vi "UV_Parameters.vi"(6 "A/M (F:auto)":bool, 7 "R/W (F:read)":bool, 8 "error in":errorcluster, 9 "param":T1, 10 "CHN":T2 items=["All", "CH1", "CH2", "CH3", "CH4"], 11 "VISA resource":refnum<visa-resource-name>) -> (0 "error out":errorcluster, 2 "chn param":u8[](array[numeric]) format="%.0x", 3 "VISA resource out":refnum<visa-resource-name>, 5 "Err?":bool)   [LabVIEW 8.6]
uses:
  TypeDef/UVLed_func.ctl
  TypeDef/UVLed_channel.ctl
panel:
  # "For Manual and Auto Mode Only"
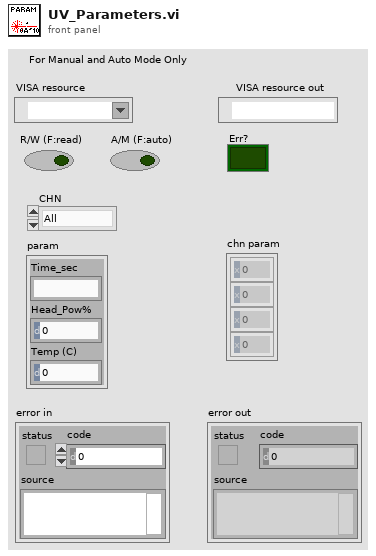
[diagram p1: front panel]
types:
  T1 = cluster{"Time_sec":string, "Head_Pow%":i32, "Temp (C)":u8}
  T2 = typedef "UVLed_channel.ctl" = u16
  T3 = typedef "UVLed_func.ctl" = u16
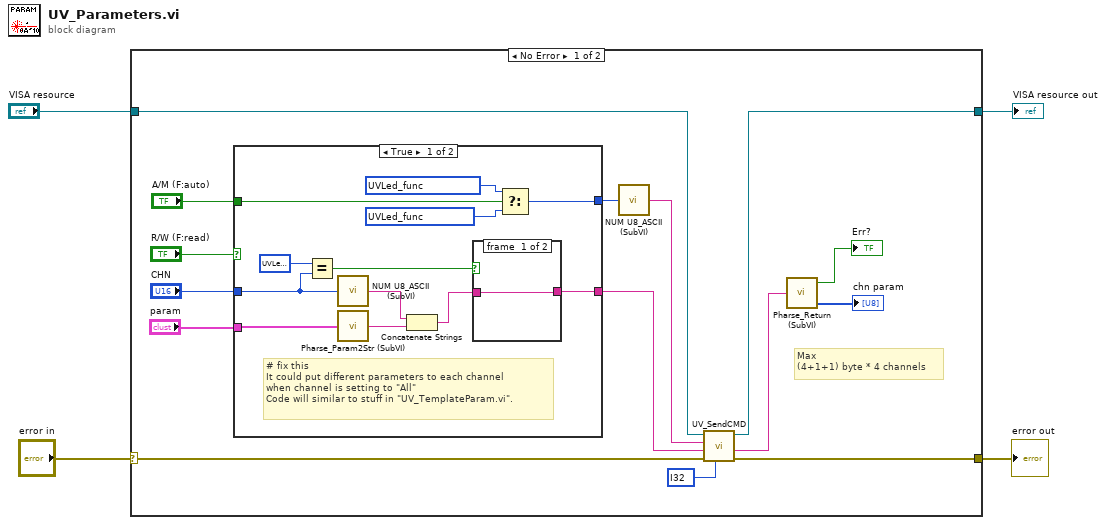
[diagram p0: block diagram]
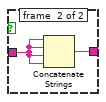
[diagram p2: hidden frame]
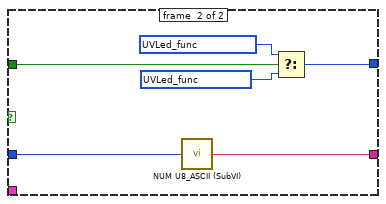
[diagram p3: hidden frame]
diagram:
  n1 = case shown="No Error" "error in" {
    selector: "error in" -> [w16 w42]
    tunnel: [w15 w42] -> w3
    tunnel: "VISA resource" -> [w17 w41]
    tunnel: [w13 w41] -> w1
    frame #0 {
      # "Max\n(4+1+1) byte * 4 channels"
      n2 = case shown="True" "R/W (F:read)" {
        tunnel: [w31 w40] -> w19
        tunnel: "A/M (F:auto)" -> [w30 w37]
        tunnel: [w22 w36] -> w10
        tunnel: "CHN" -> [w26 w35]
        tunnel: "param" -> [w21 _]
        frame #0 {
          w25 = T2 ? items=["All", "CH1", "CH2", "CH3", "CH4"] ("x")
          w28 = T3 ? items=["GetAllStatus", "LightOn", "LightOff", "AllForceOff", "GetMenuChnPara", "SetMenuChnPara", "GetAutoChnPara", "SetAutoChnPara", "GetMenuTemplate", "SetMenuTemplate", "GetAutoTemplate", "SetAutoTemplate", "GetTemplatePara", "SetTemplatePara", "GetMode", "SetMode", "ChkErr"] ("Function")
          w29 = T3 ? items=["GetAllStatus", "LightOn", "LightOff", "AllForceOff", "GetMenuChnPara", "SetMenuChnPara", "GetAutoChnPara", "SetAutoChnPara", "GetMenuTemplate", "SetMenuTemplate", "GetAutoTemplate", "SetAutoTemplate", "GetTemplatePara", "SetTemplatePara", "GetMode", "SetMode", "ChkErr"] ("Function")
          # "# fix this\nIt could put different parameters to each channel \nwhen channel is setting to \"All\"\nCode will similar to stuff in \"UV_TemplateParam.vi\"."
          n3 = Equal?(x=w25, y=w26) -> (x = y?=w23:bool)
          n4 = call "NUM U8_ASCII (SubVI).vi"("Numeric"=w26) -> ("String out"=w27:string)
          n5 = call "Pharse_Param2Str (SubVI).vi"("param"=w21) -> ("param_cmd"=w20:string)
          n6 = Concatenate Strings(w27, w20) -> (w24:string)
          n7 = case shown="True" w23 {
            tunnel: w24 -> [w32 w34]
            tunnel: [w32 w33] -> w22
            frame #0 {
            }
            frame #1 {
              n8 = Concatenate Strings(w34, w34, w34, w34) -> (w33:string)
            }
          }
          n9 = Select(t=w29, s=w30, f=w28) -> (s? t:f=w31:T3)
        }
        frame #1 {
          w38 = T3 ? items=["GetAllStatus", "LightOn", "LightOff", "AllForceOff", "GetMenuChnPara", "SetMenuChnPara", "GetAutoChnPara", "SetAutoChnPara", "GetMenuTemplate", "SetMenuTemplate", "GetAutoTemplate", "SetAutoTemplate", "GetTemplatePara", "SetTemplatePara", "GetMode", "SetMode", "ChkErr"] ("Function")
          w39 = T3 ? items=["GetAllStatus", "LightOn", "LightOff", "AllForceOff", "GetMenuChnPara", "SetMenuChnPara", "GetAutoChnPara", "SetAutoChnPara", "GetMenuTemplate", "SetMenuTemplate", "GetAutoTemplate", "SetAutoTemplate", "GetTemplatePara", "SetTemplatePara", "GetMode", "SetMode", "ChkErr"] ("Function")
          n10 = call "NUM U8_ASCII (SubVI).vi"("Numeric"=w35) -> ("String out"=w36:string)
          n11 = Select(t=w39, s=w37, f=w38) -> (s? t:f=w40:T3)
        }
      }
      n12 = call "NUM U8_ASCII (SubVI).vi"("Numeric"=w19) -> ("String out"=w18:string)
      n13 = call "UV_SendCMD.vi"("delay(ms)"=i32 ?, "error in"=w16, "value"=w10, "function"=w18, "VISA resource name"=w17) -> ("error out"=w15:errorcluster, "response"=w14:string, "VISA resource name out"=w13:refnum<visa-resource-name>)  [unwired: 4 in]
      n14 = call "Pharse_Return (SubVI).vi"("buffer in"=w14) -> ("byte array"=→"chn param":u8[], "Err?"=→"Err?":bool)  [unwired: 2 in, 1 out]
    }
    frame #1 {
    }
  }
  "error out" <- w3
  "VISA resource out" <- w1
